vi "sub_process data no queue.vi"(1 "Raw Data":dbl[](array[numeric]), 2 "Elapsed Time (s)":dbl) -> (0 "Processed Data":dbl[](array[numeric]))   [LabVIEW 2020]
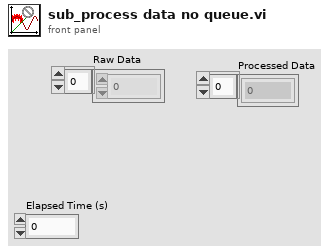
[diagram p1: front panel]
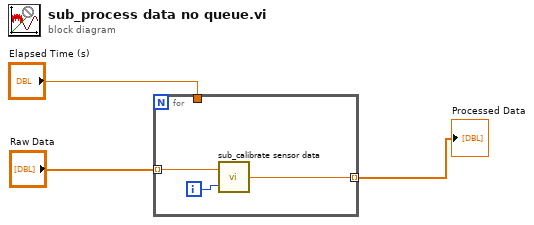
[diagram p0: block diagram]
diagram:
  n1 = for {
    tunnel: "Raw Data" -> [w5] mode=indexing
    tunnel: "Elapsed Time (s)" -> [_]
    tunnel: [w4] -> w1 mode=indexing
    i -> [w6]
    n2 = call "sub_calibrate sensor data.vi"("Sensor Column"=w6, "Raw Data"=w5) -> ("Calibrated Data"=w4:dbl)
  }
  "Processed Data" <- w1
